vi "Template.vi"   [LabVIEW 2010]
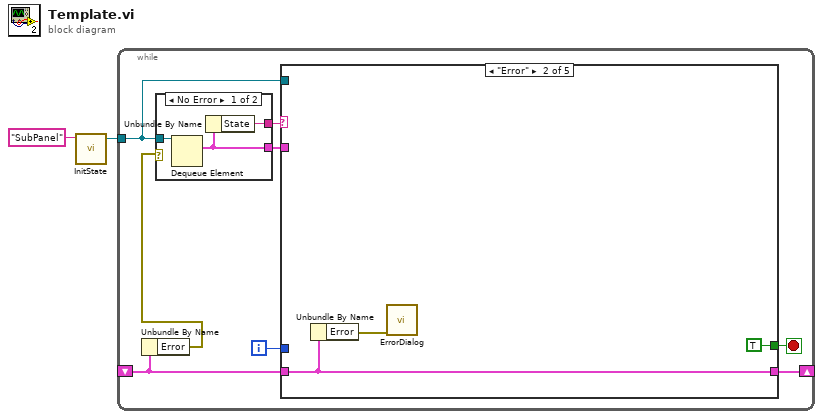
[diagram p0: block diagram]
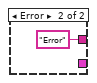
[diagram p2: hidden frame]
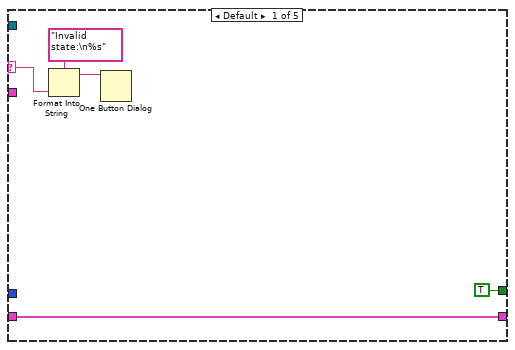
[diagram p3: hidden frame]
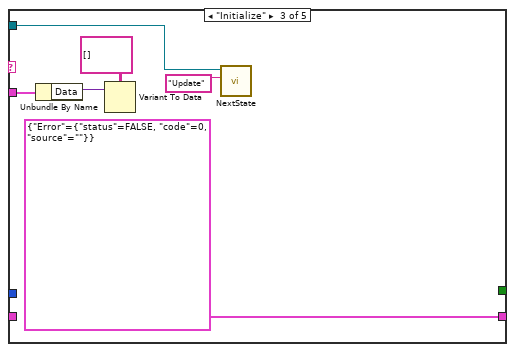
[diagram p4: hidden frame]
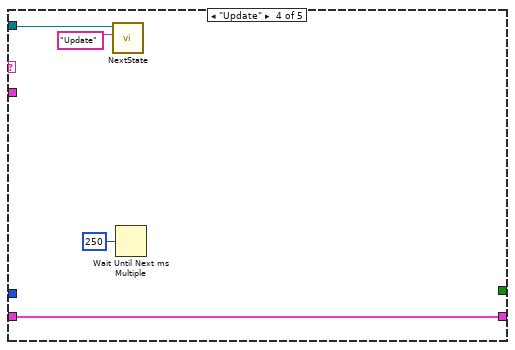
[diagram p5: hidden frame]
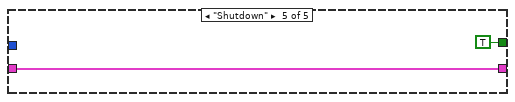
[diagram p6: hidden frame]
diagram:
  n1 = call "InitState.vi"("Name"="SubPanel" ("name (unnamed)")) -> ("Queue Out"=w2:refnum<queue>)  [unwired: 8 in, 1 out]
  n2 = while {
    tunnel: w2 -> [w8]
    shift-right: [w7] -> _
    shift-left: _ -> [w5]
    i -> [w3]
    stop <- w4 stop-if-true
    n3 = Unbundle By Name(w5) -> ("Error"=w6:errorcluster)
    n4 = case shown="No Error" w6 {
      tunnel: w8 -> [w13 _]
      tunnel: [w12 "Error" ("State")] -> w10
      tunnel: [w11 _] -> w9
      frame No Error {
        n5 = Dequeue Element(queue=w13) -> (element=w11:cluster{"State":string, "Data":variant})  [unwired: 2 in, 3 out]
        n6 = Unbundle By Name(w11) -> ("State"=w12:string)
      }
      frame Error {
      }
    }
    n7 = case shown="\"Error\"" w10 {
      selector: w10 -> [w17 _ _ _ _]
      tunnel: w9 -> [_ _ w27 _ _]
      tunnel: w8 -> [_ _ w23 w29 _]
      tunnel: [w16 w21 cluster{"Error":errorcluster} {"Error"={"status"=FALSE, "code"=0, "source"=""}} w32 w34] -> w7
      tunnel: w5 -> [w16 w21 _ w32 w34]
      tunnel: [TRUE TRUE _ _ TRUE] -> w4
      tunnel: w3 -> [_ _ _ _ _]
      frame Default {
        n8 = Format Into String(format string="Invalid state:\n%s", w17) -> (resulting string=w18:string)  [unwired: 2 in, 1 out]
        n9 = One Button Dialog(message=w18) -> ()  [unwired: 1 in, 1 out]
      }
      frame "Error" {
        n10 = Unbundle By Name(w21) -> ("Error"=w20:errorcluster)
        n11 = call "ErrorDialog.vi"("error in"=w20) -> ()  [unwired: 10 in, 1 out]
      }
      frame "Initialize" {
        n12 = Unbundle By Name(w27) -> ("Data"=w26:variant)
        n13 = Variant To Data(Variant=w26, type=string[][] [] ("subarray")) -> ()  [unwired: 1 in, 2 out]
        n14 = call "NextState.vi"("State"="Update", "Queue In"=w23) -> ()  [unwired: 8 in, 2 out]
      }
      frame "Update" {
        n15 = call "NextState.vi"("State"="Update", "Queue In"=w29) -> ()  [unwired: 8 in, 2 out]
        n16 = Wait Until Next ms Multiple(millisecond multiple=u32 250) -> ()  [unwired: 1 out]
      }
      frame "Shutdown" {
      }
    }
  }
